vi "styledtext.vi"() -> ()   [LabVIEW 2020]
panel:
  in  "numeric":dbl
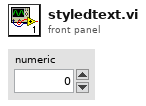
[diagram p1: front panel]
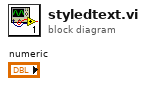
[diagram p0: block diagram]
diagram:
